vi "Table, Initialize.vi"(6 "Delete Row Headers (T)":bool=TRUE, 7 "Enable (T)":bool=TRUE, 8 "error in":errorcluster, 9 "column_n (0)":i32, 10 "row_n (0)":i32, 11 "Tbl Refnum":refnum<vi>) -> (0 "error out":errorcluster, 3 "Tbl Refnum dup":refnum<vi>)   [LabVIEW 2010]
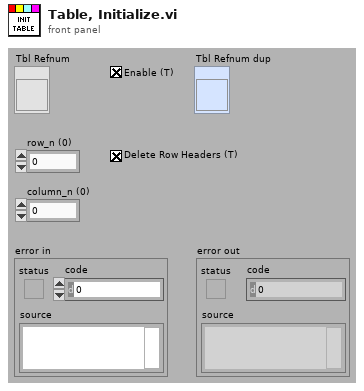
[diagram p1: front panel]
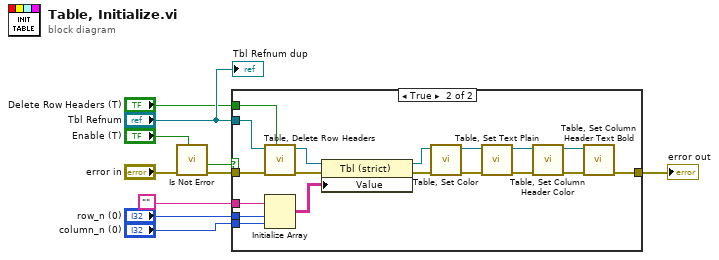
[diagram p0: block diagram]
diagram:
  n1 = call "Is Not Error.vi"("enable (T)"="Enable (T)", "error in"="error in") -> ("error out"=w2:errorcluster, "ready"=w1:bool)  [unwired: 4 in, 1 out]
  n2 = case shown="True" w1 {
    tunnel: [w11 w16] -> w10
    tunnel: "row_n (0)" -> [_ w27]
    tunnel: "column_n (0)" -> [_ w26]
    tunnel: "" -> [_ w25]
    tunnel: "Tbl Refnum" -> [_ w22]
    tunnel: "Delete Row Headers (T)" -> [_ w21]
    tunnel: w2 -> [w11 w19]
    frame False {
    }
    frame True {
      n3 = call "Table, Delete Row Headers.vi"("Enable (T)"=w21, "error in"=w19, "Tbl Refnum"=w22) -> ("error out"=w24:errorcluster, "Tbl Refnum dup"=w23:refnum<vi>)  [unwired: 7 in]
      n4 = Initialize Array(w25, w27, w26) -> (w29:string[][])
      n5 = property class="Tbl (strict)"(reference=w23, error in=w24, "Value"=w29) -> (reference out=w20:refnum<vi>, error out=w28:errorcluster)
      n6 = call "Table, Set Color.vi"("error in"=w28, "Tbl Refnum"=w20) -> ("error out"=w18:errorcluster, "Tbl Refnum out"=w17:refnum<vi>)  [unwired: 7 in]
      n7 = call "Table, Set Text Plain.vi"("error in"=w18, "Tbl Refnum"=w17) -> ("error out"=w15:errorcluster, "Tbl Refnum out"=w13:refnum<vi>)  [unwired: 6 in]
      n8 = call "Table, Set Column Header Color.vi"("error in"=w15, "Tbl Refnum"=w13) -> ("error out"=w14:errorcluster, "Tbl Refnum out"=w12:refnum<vi>)  [unwired: 6 in]
      n9 = call "Table, Set Column Header Text Bold.vi"("error in"=w14, "Tbl Refnum"=w12) -> ("error out"=w16:errorcluster)  [unwired: 6 in, 1 out]
    }
  }
  "error out" <- w10
  "Tbl Refnum dup" <- "Tbl Refnum"
